vi "Global Variables.vi"() -> ()   [LabVIEW 2017]
panel:
  in  "Quit?":bool
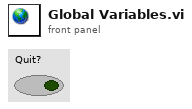
[diagram p1: front panel]
diagram:
